vi "Query instrument.vi"(8 "error in (no error)":errorcluster, 10 "Command":string="vlimit?\n", 11 "COM port in":refnum<visa-resource-name>) -> (0 "error out":errorcluster, 2 "read buffer":string, 3 "COM port out":refnum<visa-resource-name>)   [LabVIEW 2020]
uses:
  00f5608b-1276-4cf8-b19d-5f402c4248f9.vi
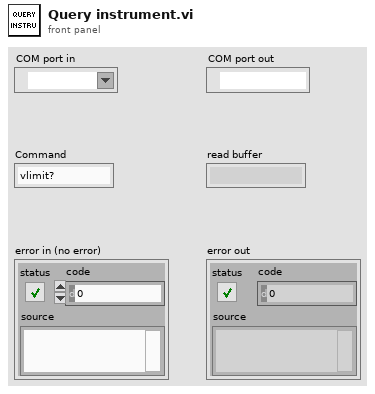
[diagram p1: front panel]
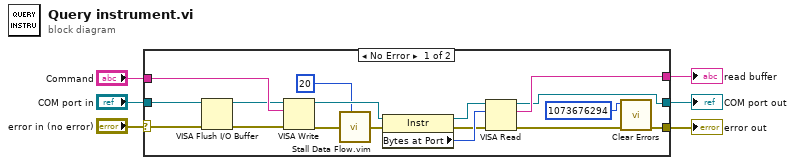
[diagram p0: block diagram]
diagram:
  n1 = case shown="No Error" "error in (no error)" {
    selector: "error in (no error)" -> [w13 w25]
    tunnel: [w10 w25] -> w6
    tunnel: [w23 _] -> w5
    tunnel: [w22 w24] -> w4
    tunnel: "Command" -> [w14 _]
    tunnel: "COM port in" -> [w8 w24]
    frame No Error {
      n2 = VISA Flush I/O Buffer(VISA resource name=w8, error in (no error)=w13) -> (VISA resource name out=w7:refnum<visa-resource-name>, error out=w9:errorcluster)  [unwired: 1 in]
      n3 = VISA Write(VISA resource name=w7, write buffer=w14, error in (no error)=w9) -> (VISA resource name out=w19:refnum<visa-resource-name>, error out=w15:errorcluster)  [unwired: 1 out]
      n4 = call "Stall Data Flow.vim"("value in"=w15, "milliseconds to wait"=u32 20) -> ("value out"=w17:errorcluster)  [unwired: 1 out]
      n5 = property class="Instr"(reference=w19, error in=w17) -> (reference out=w21:refnum<visa-resource-name>, error out=w18:errorcluster, "Bytes at Port"=w20:u32)
      n6 = VISA Read(VISA resource name=w21, byte count=w20, error in (no error)=w18) -> (VISA resource name out=w22:refnum<visa-resource-name>, read buffer=w23:string, error out=w11:errorcluster)  [unwired: 1 out]
      n7 = call <vilib>:"Clear Errors.vi"("error in (no error)"=w11, "specific error code to clear (0: all)"=1073676294) -> ("error out"=w10:errorcluster)  [unwired: 4 in, 1 out]
    }
    frame Error {
    }
  }
  "error out" <- w6
  "read buffer" <- w5
  "COM port out" <- w4
